vi "calc_lifetime.vi"(1 "error in":errorcluster, 2 "unbinned data":u16[][](array[numeric])) -> (0 "lifetimes":sgl[](array[numeric]))   [LabVIEW 2013]
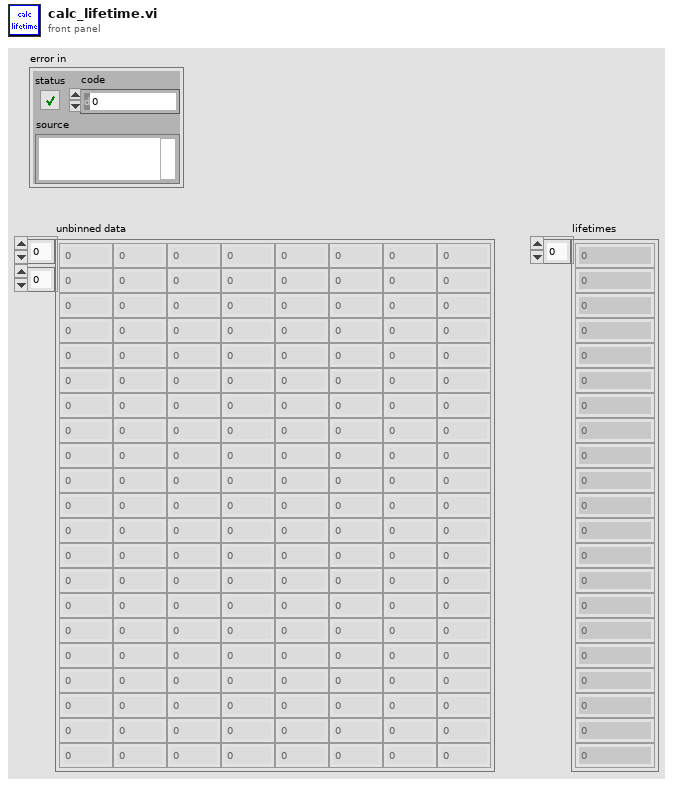
[diagram p1: front panel]
types:
  T1 = cluster{"Z_n":i32[], "devidx":i32, "initialized":bool, "acq time":i32, "Bin size":enum16{"1", "2", "4", "8", "16", "32", "64", "128"}, "# bins":i32, "sync rate":i32, "truncate":bool, "Ch0 Level":i32, "Ch1 Level":i32, "Ch0 ZeroX":i32, "Ch1 ZeroX":i32, "resolution":i32}
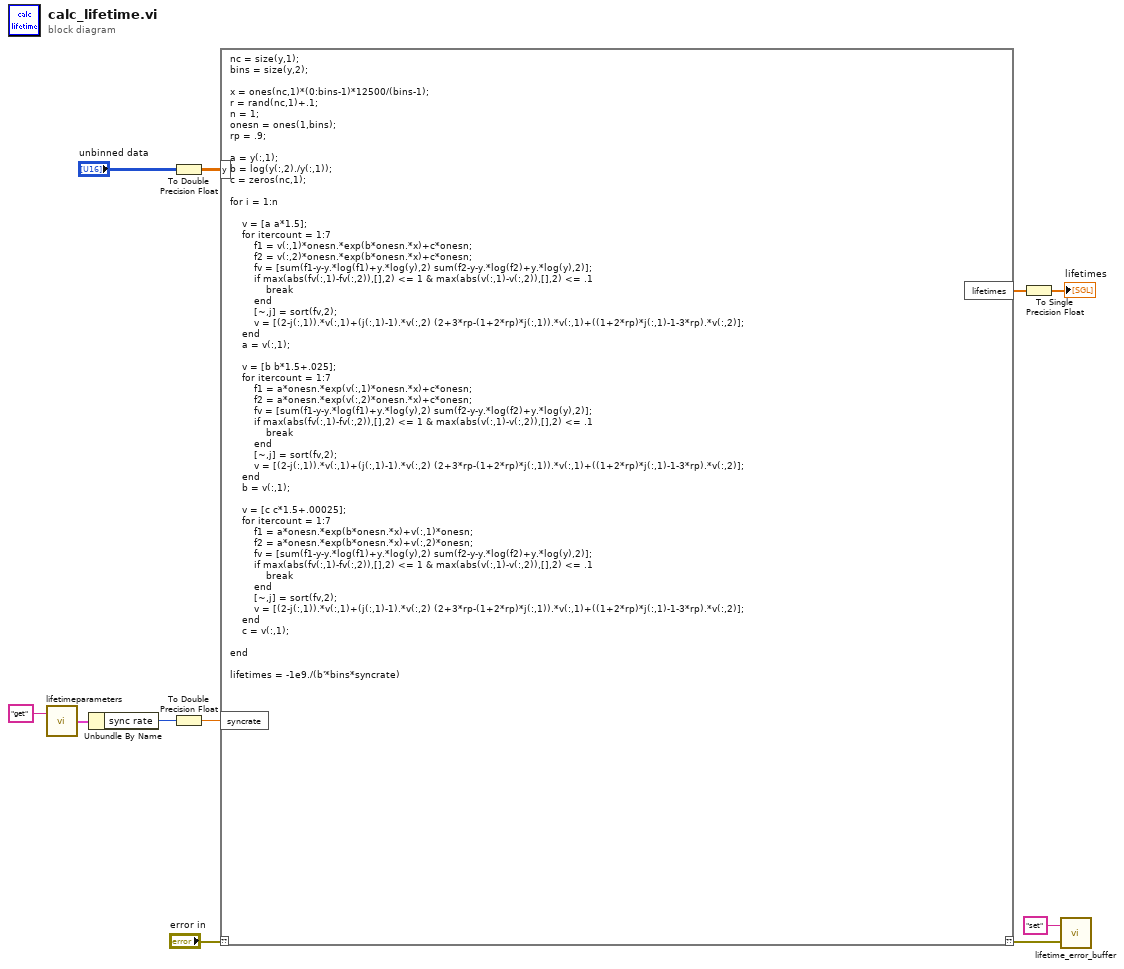
[diagram p0: block diagram]
diagram:
  n1 = call "lifetimeparameters.vi"("command"="get") -> ("Params out"=w11:T1)  [unwired: 1 in]
  n2 = Unbundle By Name(w11) -> ("sync rate"=w9:i32)
  n3 = To Double Precision Float(number="unbinned data") -> (double precision float=w6:dbl[][])
  n4 = To Double Precision Float(number=w9) -> (double precision float=w4:dbl)
  n5 = script code="nc = size(y,1);\nbins = size(y,2);\n\nx = ones(nc,1)*(0:bins-1)*12500/(bins-1);\nr = rand(nc,1)+.1;\nn = 1;\nonesn = ones(1,bins);\nrp = .9;\n\na = y(:,1);\nb = log(y(:,2)./y(:,1));\nc = zeros(nc,1);\n\nfor i = 1:n\n    \n    v = [a a*1.5];\n    for itercount = 1:7    \n        f1 = v(:,1)*onesn.*exp(b*onesn.*x)+c*onesn;\n        f2 = v(:,2)*onesn.*exp(b*onesn.*x)+c*onesn;\n        fv = [sum(f1-y-y.*log(f1)+y.*log(y),2) sum(f2-y-y.*log(f2)+y.*log(y),2)];\n        if max(abs(fv(:,1)-fv(:,2)),[],2) <= 1 & max(abs(v(:,1)-v(:,2)),[],2) <= .1\n            break\n        end\n        [~,j] = sort(fv,2); \n        v = [(2-j(:,1)).*v(:,1)+(j(:,1)-1).*v(:,2) (2+3*rp-(1+2*rp)*j(:,1)).*v(:,1)+((1+2*rp)*j(:,1)-1-3*rp).*v(:,2)];\n    end\n    a = v(:,1);\n    \n    v = [b b*1.5+.025]; \n    for itercount = 1:7\n        f1 = a*onesn.*exp(v(:,1)*onesn.*x)+c*onesn;\n        f2 = a*onesn.*exp(v(:,2)*onesn.*x)+c*onesn;\n        fv = [sum(f1-y-y.*log(f1)+y.*log(y),2) sum(f2-y-y.*log(f2)+y.*log(y),2)];\n        if max(abs(fv(:,1)-fv(:,2)),[],2) <= 1 & max(abs(v(:,1)-v(:,2)),[],2) <= .1\n            break\n        end\n        [~,j] = sort(fv,2); \n        v = [(2-j(:,1)).*v(:,1)+(j(:,1)-1).*v(:,2) (2+3*rp-(1+2*rp)*j(:,1)).*v(:,1)+((1+2*rp)*j(:,1)-1-3*rp).*v(:,2)];\n    end\n    b = v(:,1);\n    \n    v = [c c*1.5+.00025]; \n    for itercount = 1:7\n        f1 = a*onesn.*exp(b*onesn.*x)+v(:,1)*onesn;\n        f2 = a*onesn.*exp(b*onesn.*x)+v(:,2)*onesn;\n        fv = [sum(f1-y-y.*log(f1)+y.*log(y),2) sum(f2-y-y.*log(f2)+y.*log(y),2)];\n        if max(abs(fv(:,1)-fv(:,2)),[],2) <= 1 & max(abs(v(:,1)-v(:,2)),[],2) <= .1\n            break\n        end\n        [~,j] = sort(fv,2); \n        v = [(2-j(:,1)).*v(:,1)+(j(:,1)-1).*v(:,2) (2+3*rp-(1+2*rp)*j(:,1)).*v(:,1)+((1+2*rp)*j(:,1)-1-3*rp).*v(:,2)];\n    end\n    c = v(:,1);\n    \nend\n\nlifetimes = -1e9./(b'*bins*syncrate)"("??"="error in", "y"=w6, "syncrate"=w4) -> ("??"=w2:errorcluster, "lifetimes"=w5:dbl[])
  n6 = To Single Precision Float(number=w5) -> (single precision float=→"lifetimes":sgl[])
  n7 = call "lifetime_error_buffer.vi"("error in"=w2, "command"="set") -> ()  [unwired: 1 out]
